vi "PrepareListBoxFromDropletDB.vi"(8 "error in (no error)":errorcluster, 10 "Reference to Listbox":refnum<vi>, 11 "DropletDBListBoxCtl":T1) -> (0 "error out":errorcluster)   [LabVIEW 2013]
doc: "Use this template to build a VI to use as a subVI."
uses:
  TypeDef/DropletDBListBox.ctl
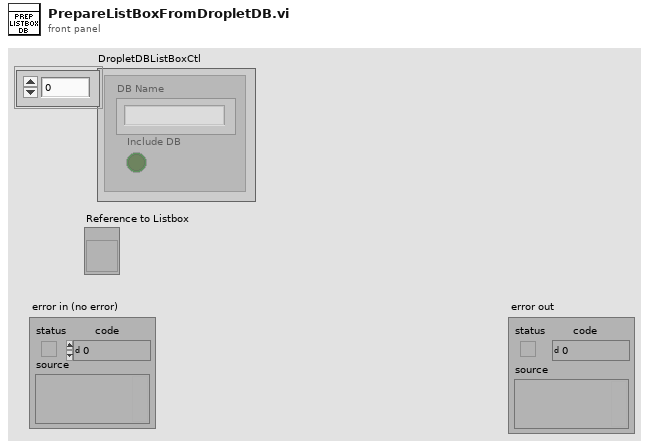
[diagram p1: front panel]
types:
  T1 = typedef "DropletDBListBox.ctl" = cluster{"DB Name":string, "Include DB":bool}[]
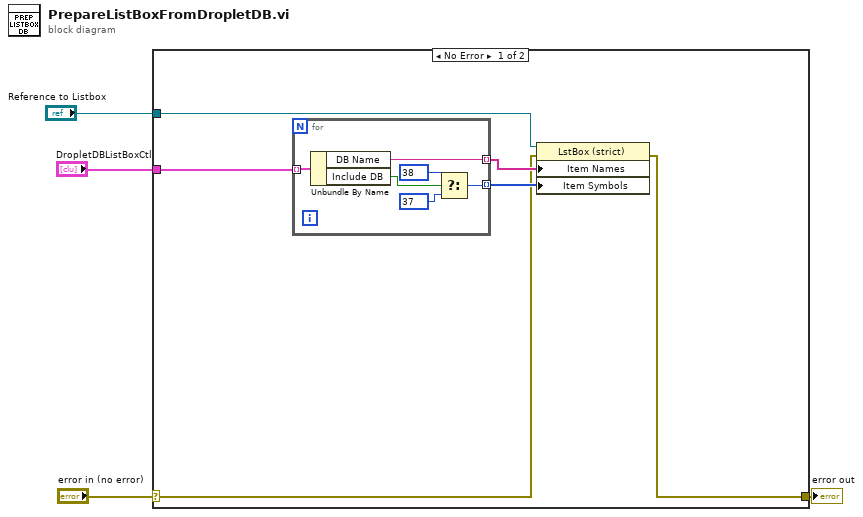
[diagram p0: block diagram]
diagram:
  n1 = case shown="No Error" "error in (no error)" {
    selector: "error in (no error)" -> [w6 w17]
    tunnel: [w5 w17] -> w3
    tunnel: "DropletDBListBoxCtl" -> [w10 _]
    tunnel: "Reference to Listbox" -> [w7 _]
    frame No Error {
      n2 = for {
        tunnel: w10 -> [w16] mode=indexing
        tunnel: [w15] -> w9 mode=indexing
        tunnel: [w13] -> w8 mode=indexing
        n3 = Unbundle By Name(w16) -> ("DB Name"=w15:string, "Include DB"=w14:bool)
        n4 = Select(t=38 ("Item Symbols"), s=w14, f=37 ("Item Symbols")) -> (s? t:f=w13:i32)
      }
      n5 = property on="Property Node" class="LstBox (strict)"(reference=w7, error in=w6, "Item Names"=w9, "Item Symbols"=w8) -> (error out=w5:errorcluster)  [unwired: 1 out]
    }
    frame Error {
    }
  }
  "error out" <- w3
